vi "myRIO_BRig_RT_dataTrial_Time.vi"() -> (2 "output_Time":i32)   [LabVIEW 2014]
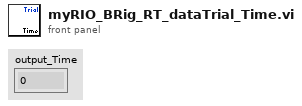
[diagram p1: front panel]
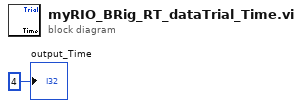
[diagram p0: block diagram]
diagram:
  "output_Time" <- 4 ("output_iBlock")
